vi "windowTD.vi"(4 "Divisor (conversion factor between units)":dbl format="%.2f", 5 "Graph Ref":refnum<vi>, 6 "MatrixSize":u32, 7 "Matrix Selected":i32, 8 "Units":enum16{"PM", "GHz"}(ring), 9 "Sigma (ns)":dbl format="%.3f", 10 "x2 (ns or m)":dbl format="%.2f", 11 "x1 (ns or m)":dbl format="%.2f") -> (2 "Res. BW":dbl=838.8608 caption="Window Res BW (pm)" format="%.2f", 3 "Windowed JM Cluster":cluster{dbl, "time inc (ns)_":dbl, dbl[][]} {"?" format="%.2f"; "time inc (ns)_" format="%.6f"; "?" format="%.2f"})   [LabVIEW 2012]
uses:
  bin/OVA32.dll
panel:
  out "timeInc":dbl format="%.6f"
  # "Max value in time domain"
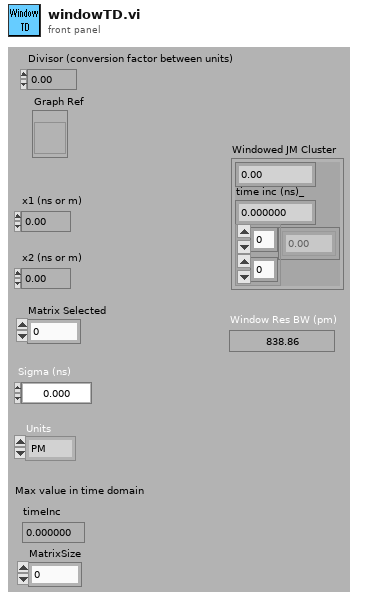
[diagram p1: front panel]
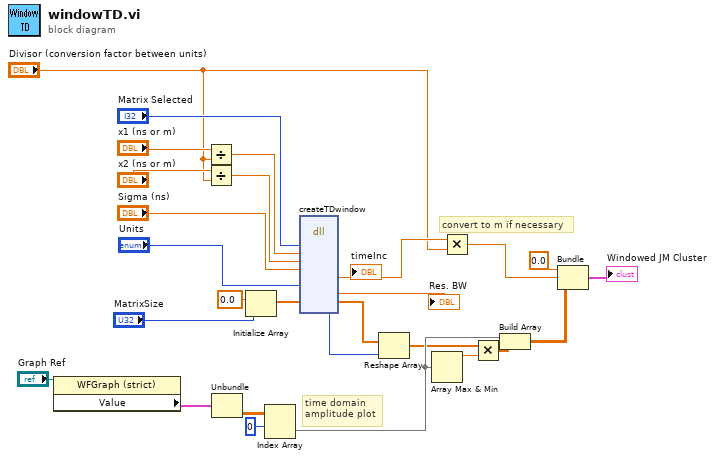
[diagram p0: block diagram]
diagram:
  # "time domain \namplitude plot"
  # "convert to m if necessary"
  n1 = property class="WFGraph (strict)"(reference="Graph Ref") -> ("Value"=w12:cluster{"X0":dbl, "dX":dbl, "Data":dbl[][]})  [unwired: 1 in, 2 out]
  n2 = Divide(x="x1 (ns or m)", y="Divisor (conversion factor between units)") -> (x/y=w14:dbl)
  n3 = Divide(x="x2 (ns or m)", y="Divisor (conversion factor between units)") -> (x/y=w15:dbl)
  n4 = Unbundle(w12) -> ("Data"=w11:dbl[][])  [unwired: 2 out]
  n5 = Initialize Array(0.0 ("Element Data"), "MatrixSize") -> (w3:dbl[])
  n6 = Index Array(array=w11, index (row)=0 ("Index (row)")) -> (element=w8:dbl[])  [unwired: 1 in]
  n7 = dll-call lib="C:/_src/OVA5000_DSP_falcon/Software/LabVIEW/OVA/SDK/OVA_5000_SDK_v5.14.3/bin/OVA32.dll" fn="createTDwindow"("matrix"="Matrix Selected", "curosor1"=w14, "cursor2"=w15, "sigma"="Sigma (ns)", "uints"="Units", "windowTD"=w3) -> ("timeInc"=w19:dbl, "windRSBW"=→"Res. BW":dbl, "windowTD"=w21:dbl[], "windowSize"=w5:u32)  [unwired: 12 in, 2 out]
  "timeInc" <- w19
  n8 = Reshape Array(w21, w5) -> (w7:dbl[])
  n9 = Array Max & Min(array=w8) -> (max value=w9:dbl)  [unwired: 3 out]
  n10 = Multiply(x=w19, y="Divisor (conversion factor between units)") -> (x*y=w20:dbl)
  n11 = Multiply(x=w7, y=w9) -> (x*y=w6:dbl[])
  n12 = Build Array(w8, w6) -> (w23:dbl[][])
  n13 = Bundle(0.0, w20, w23) -> (→"Windowed JM Cluster":cluster{dbl, dbl, dbl[][]})  [unwired: 1 in]
